vi "StepDeploy Test.vi"(11 "Pilot-CoPilot Gamepad Controls":T1) -> ()   [LabVIEW 2014]
uses:
  Subsystems VIs/Robot Control Outputs 2015.ctl
  <vilib>/Rock Robotics/WPI/Solenoid/WPI_SolenoidValue.ctl
  Global Variables/Refnum Names.vi
  <vilib>/Rock Robotics/WPI/Solenoid/WPI_SolenoidSetEnum.vi
panel:
  # "CB = control board"
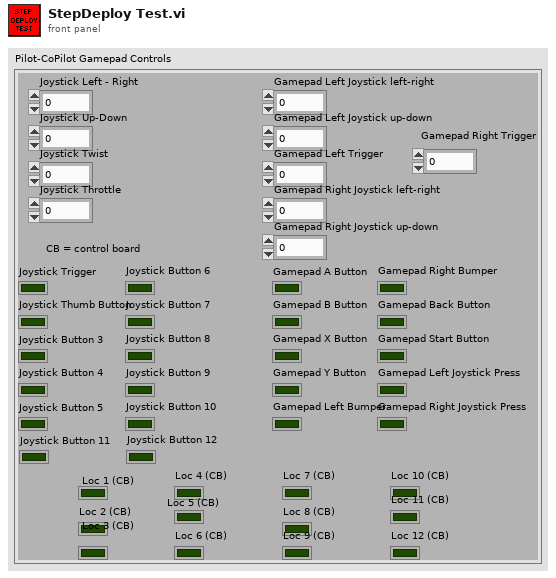
[diagram p1: front panel]
types:
  T1 = typedef "Robot Control Outputs 2015.ctl" = cluster{"Gamepad Left Joystick left-right":dbl, "Gamepad Left Joystick up-down":dbl, "Gamepad A Button":bool, "Gamepad B Button":bool, "Gamepad X Button":bool, "Gamepad Y Button":bool, "Gamepad Left Bumper":bool, "Gamepad Right Bumper":bool, "Gamepad Back Button":bool, "Gamepad Start Button":bool, "Gamepad Left Joystick Press":bool, "Gamepad Right Joystick Press":bool, "Joystick Trigger":bool, "Joystick Thumb Button":bool, "Joystick Button 3":bool, "Joystick Button 4":bool, "Joystick Button 5":bool, "Joystick Button 6":bool, "Joystick Button 7":bool, "Joystick Button 8":bool, "Joystick Button 9":bool, "Joystick Button 10":bool, "Gamepad Left Trigger":dbl, "Gamepad Right Joystick left-right":dbl, "Gamepad Right Joystick up-down":dbl, "Joystick Left - Right":dbl, "Joystick Up-Down":dbl, "Joystick Twist":dbl, "Joystick Throttle":dbl, "Loc 1 (CB)":bool, "Loc 4 (CB)":bool, "Gamepad Right Trigger":dbl, "Loc 2 (CB)":bool, "Loc 3 (CB)":bool, "Loc 5 (CB)":bool, "Loc 6 (CB)":bool, "Loc 7 (CB)":bool, "Loc 10 (CB)":bool, "Loc 8 (CB)":bool, "Loc 9 (CB)":bool, "Loc 11 (CB)":bool, "Loc 12 (CB)":bool, "Joystick Button 11":bool, "Joystick Button 12":bool}
  T2 = typedef "WPI_SolenoidDevRef.ctl" = cluster{"DevStatus":errorcluster, "Pneumatics Control Module":u8, "Forward Solenoid Channel":T3, "Reverse Solenoid Channel":T3}
  T3 = typedef "WPI_SolenoidChannel.ctl" = enum8{"Solenoid 0", "Solenoid 1", "Solenoid 2", "Solenoid 3", "Solenoid 4", "Solenoid 5", "Solenoid 6", "Solenoid 7", "Invalid"}
  T4 = typedef "WPI_SolenoidValue.ctl" = enum16{"Off", "On", "Forward", "Reverse"}
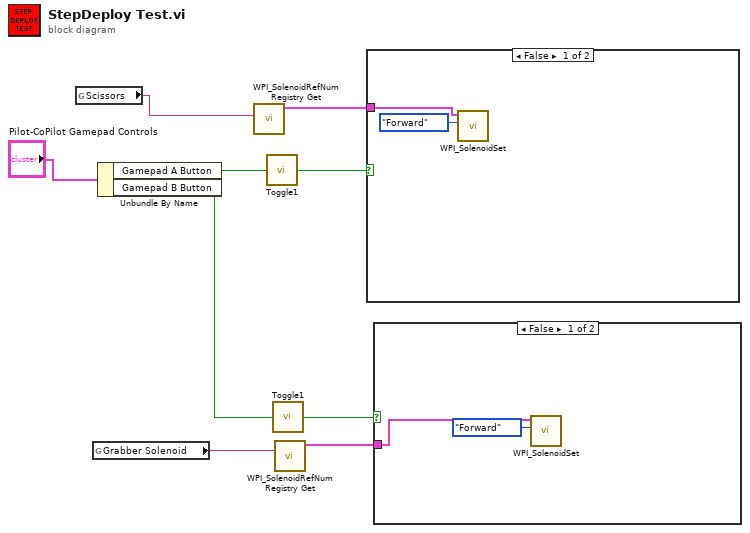
[diagram p0: block diagram]
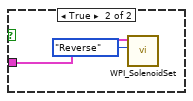
[diagram p2: hidden frame]
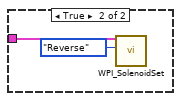
[diagram p3: hidden frame]
diagram:
  n1 = global read "Refnum Names.vi" "Scissors"() -> (w5:string)
  n2 = global read "Refnum Names.vi" "Grabber Solenoid"() -> (w4:string)
  n3 = Unbundle By Name("Pilot-CoPilot Gamepad Controls") -> ("Gamepad A Button"=w8:bool, "Gamepad B Button"=w2:bool)
  n4 = call <vilib>:"WPI_SolenoidRefNum Registry Get.vi"("refnum name"=w5) -> ("SolenoidDevRef"=w6:T2)  [unwired: 9 in, 1 out]
  n5 = call "Toggle1.vi"("Boolean"=w8) -> ("Driver Switch 2"=w7:bool)
  n6 = call "Toggle1.vi"("Boolean"=w2) -> ("Driver Switch 2"=w1:bool)
  n7 = call <vilib>:"WPI_SolenoidRefNum Registry Get.vi"("refnum name"=w4) -> ("SolenoidDevRef"=w3:T2)  [unwired: 9 in, 1 out]
  n8 = case shown="False" w7 {
    tunnel: w6 -> [w11 w13]
    frame False {
      n9 = call-poly <vilib>:"WPI_SolenoidSet.vi"("Value"=WPI_SolenoidValue."Forward", "SolenoidDevRef"=w11) -> ()  [unwired: 8 in, 2 out]
    }
    frame True {
      n10 = call-poly <vilib>:"WPI_SolenoidSet.vi"("Value"=WPI_SolenoidValue."Reverse", "SolenoidDevRef"=w13) -> ()  [unwired: 8 in, 2 out]
    }
  }
  n11 = case shown="False" w1 {
    tunnel: w3 -> [w15 w17]
    frame False {
      n12 = call-poly <vilib>:"WPI_SolenoidSet.vi"("Value"=WPI_SolenoidValue."Forward", "SolenoidDevRef"=w15) -> ()  [unwired: 8 in, 2 out]
    }
    frame True {
      n13 = call-poly <vilib>:"WPI_SolenoidSet.vi"("Value"=WPI_SolenoidValue."Reverse", "SolenoidDevRef"=w17) -> ()  [unwired: 8 in, 2 out]
    }
  }
